vi "getTimeFromFileName.vi"(8 "errorIn":errorcluster, 11 "fileName":string) -> (0 "errorOut":errorcluster, 3 "date":dbl)   [LabVIEW 2025]
uses:
  <vilib>/regexp/Match Regular Expression.xnode
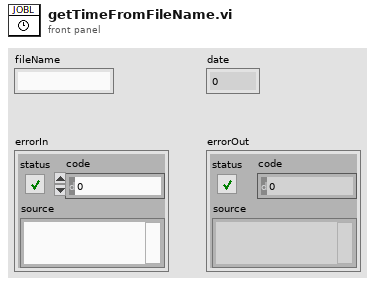
[diagram p1: front panel]
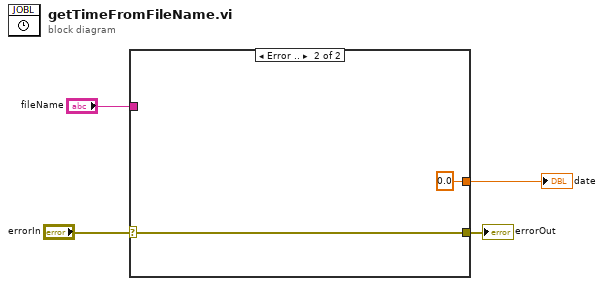
[diagram p0: block diagram]
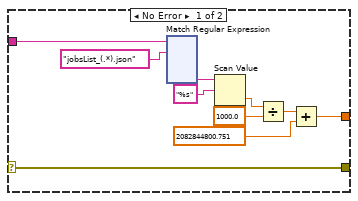
[diagram p2: hidden frame]
diagram:
  n1 = case shown="Error .." "errorIn" {
    selector: "errorIn" -> [w5 w135]
    tunnel: "fileName" -> [w12 _]
    tunnel: [w10 0.0] -> w3
    tunnel: [w5 w135] -> w1
    frame No Error {
      n2 = xnode "Match Regular Expression"("input string"=w12, "regular expression"="jobsList_(.*).json") -> ("submatch 1"=w14:string)  [unwired: 4 in, 5 out]
      n3 = Scan Value(string=w14, format string="%s") -> (value=w6:dbl)  [unwired: 1 in, 1 out]
      n4 = Divide(x=w6, y=1000.0) -> (x/y=w9:dbl)
      n5 = Add(x=w9, y=2082844800.751 ("x-y")) -> (x+y=w10:dbl)
    }
    frame Error {
    }
  }
  "date" <- w3
  "errorOut" <- w1
